vi "DataTranslation.vi"() -> (0 "error out":errorcluster)   [LabVIEW 2022 SP3]
uses:
  Sub_vis/Upload Data.ctl
  Globals/Meas_global.vi
  Data_Translation/Low levels/DtAinContinuous Folder/PolySubVIs/DtCreateAinChan.vi
  Data_Translation/Low levels/DtAinContinuous Folder/PolySubVIs/DtOLTimingSetInput.vi
  Data_Translation/Low levels/DtAinContinuous Folder/PolySubVIs/DtOLReadMultiple2D.vi
panel:
  out "Channels":string="0"
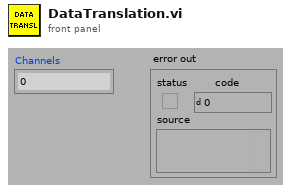
[diagram p1: front panel]
types:
  T1 = typedef "Analysis_info_cluster.ctl" = cluster{"Colour":u32, "Inst type":T2, "Inst name":string, "Symbol":string, "Code name":string, "Extra Info":string, "Inst Array":T3, "Extra Titles":string[], "Extra Values":string[], "U":dbl, "u^2":dbl, "u^3":dbl, "u^4":dbl, "Skew_u":dbl, "Kurt_u":dbl, "Sd Error in Mean":dbl, "% u'/U":dbl, "X":dbl, "Y":dbl, "Z":dbl, "Timescale integral Estimate":dbl, "Sd Error in Variance":dbl, "Calib File":path, "Calib Constants":dbl[], "Output Position":bool, "Stats":enum16{"None", "Basic", "Full"}, "Av Sampling Rate":dbl, "Av No of Samples":dbl, "Total Meas Time (s)":dbl, "ADAM Ch Name":string, "Max value":dbl, "Min value":dbl, "Req Sample Rate Hz":dbl, "Sync Delay Time (s)":dbl, "Ch No":i16, "Device":string, "Use Latest Calib":bool, "Port":string, "Metadata Ch Names":string[], "Metadata Ch Values":string[], "Label":string}
  T2 = typedef "Inst_type.ctl" = enum16{"Raw voltage", "Raw with zero offsetting", "Propeller anemometer", "Pressure Transducer", "Pitot-static tube", "Hot wire", "Cross wire 1", "Cross wire 2", "Generic Linear", "Generic Polynomial", "Generic BackPoly", "Fast FID", "Thermocouple", "Cold wire", "Pulsed Wire", "LDA Vel", "LDA Tran time", "LDA Arr time", "Microphone"}
  T3 = typedef "Instrument_Array.ctl" = enum16{"PWA", "LDA", "Analogue"}
  T4 = typedef "Device ID port info.ctl" = cluster{"Ch No":i16[], "Req Sampling Rate":dbl[], "Port":string, "Index":i32[]}
  T5 = typedef "Upload Data.ctl" = enum16{"Voltage Array", "Time Trace Cluster"}
  T6 = typedef "Setup.ctl" = enum16{"Run Program", "Show Setup", "Save Current Setup", "Setup Front Panel"}
  T7 = typedef "Rendezvous RefNum" = refnum<k1>
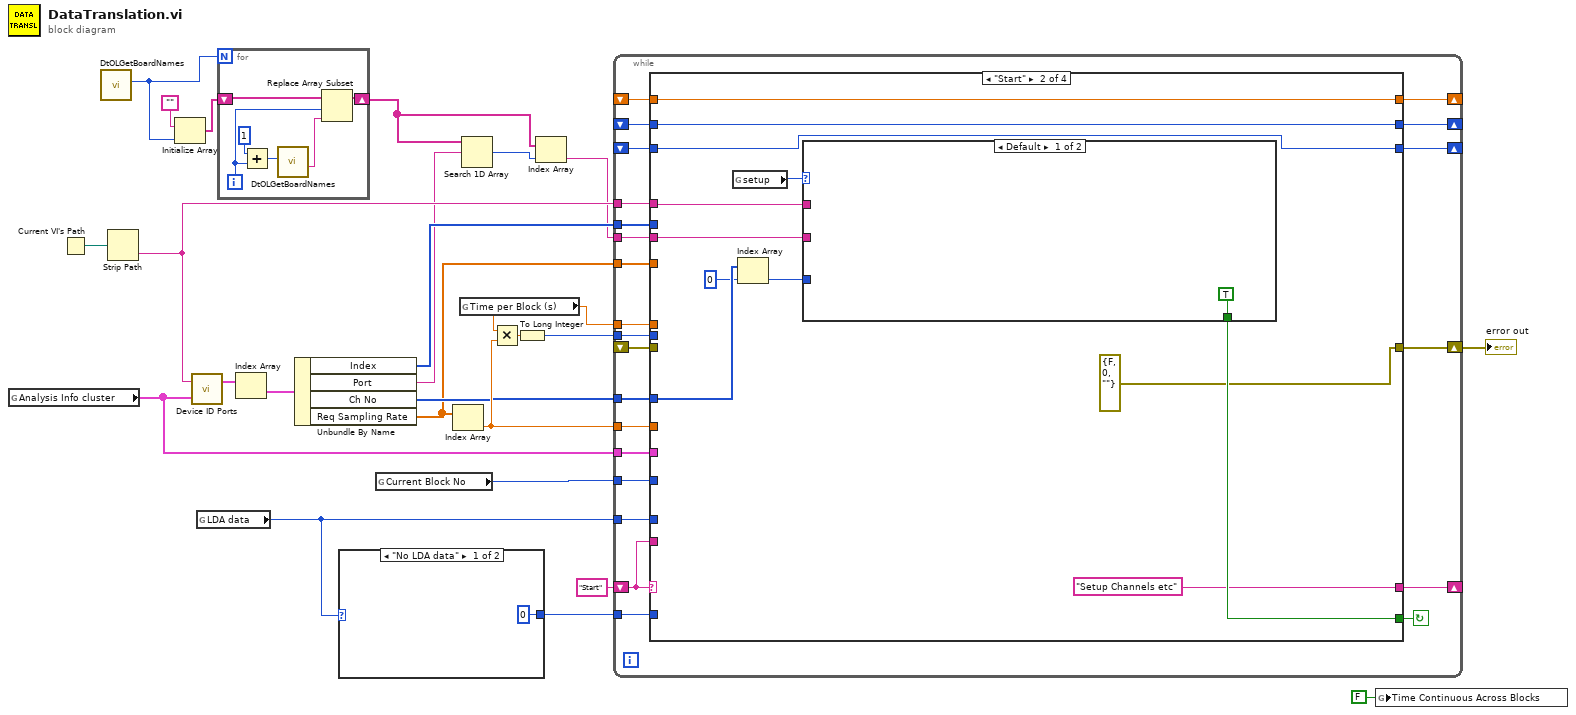
[diagram p0: block diagram]
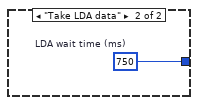
[diagram p2: hidden frame]
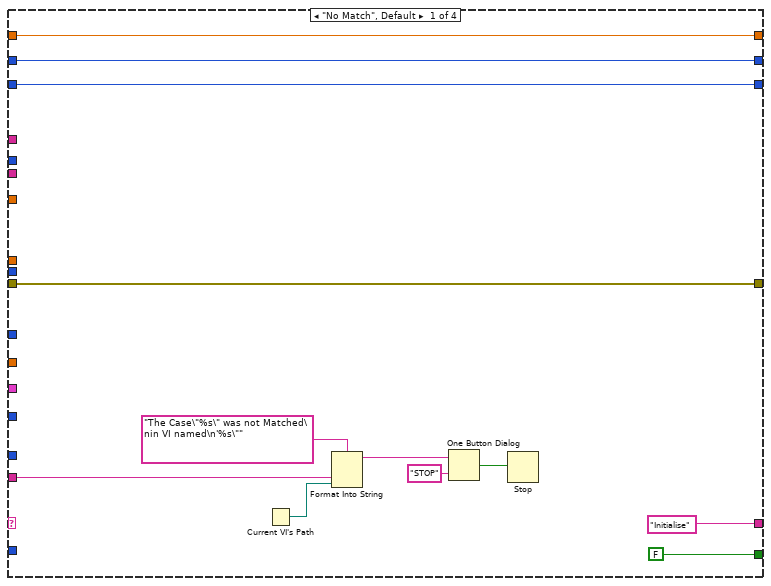
[diagram p3: hidden frame]
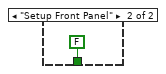
[diagram p4: hidden frame]
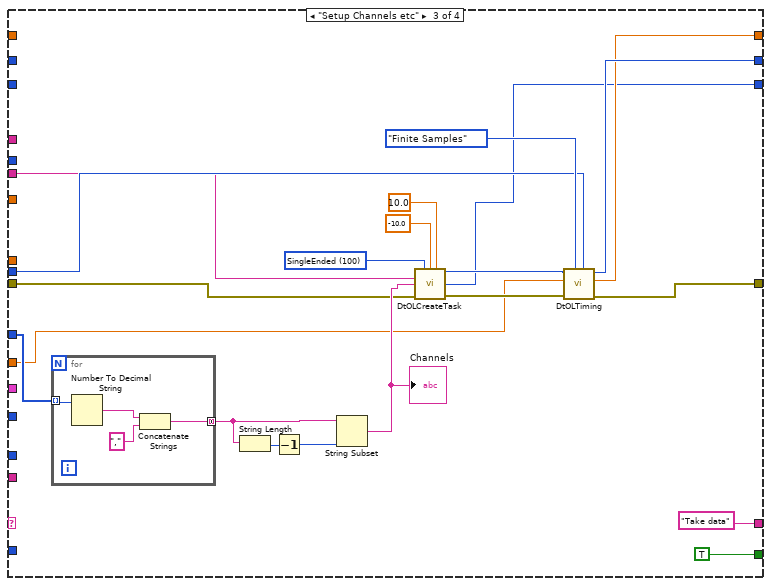
[diagram p5: hidden frame]
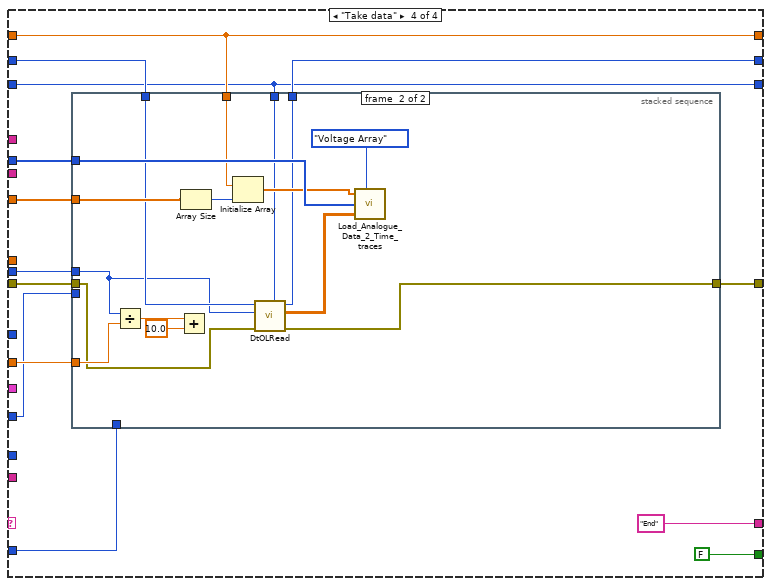
[diagram p6: hidden frame]
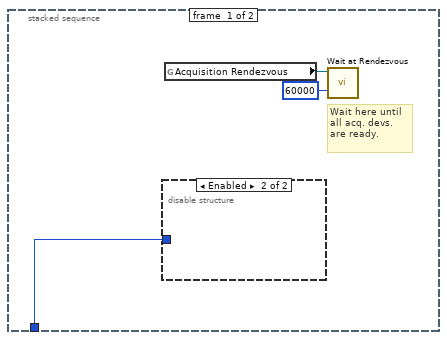
[diagram p7: hidden frame]
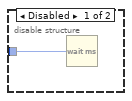
[diagram p8: hidden frame]
diagram:
  n1 = global read "Meas_global.vi" "Analysis Info cluster"() -> (w11:T1[])
  n2 = Current VI's Path() -> (path=w19:path)
  n3 = call "DtOLGetBoardNames.vi"() -> ("Number of boards"=w7:u32)  [unwired: 9 in, 2 out]
  n4 = Strip Path(path=w19) -> (name=w12:string)  [unwired: 1 out]
  n5 = Initialize Array("", w7) -> (w5:string[])
  n6 = call "Device ID Ports.vi"("Analysis Info cluster"=w11, "Device ID"=w12) -> ("Device port info"=w17:T4[])  [unwired: 1 out]
  n7 = global read "Meas_global.vi" "LDA data"() -> (w24:enum16{"No LDA data", "Take LDA data"})
  n8 = for {
    N: w7 -> [_]
    shift-right: [w28] -> w2
    shift-left: w5 -> [w29]
    i -> [w27]
    n9 = Add(x=1, y=w27) -> (x+y=w31:i32)
    n10 = call "DtOLGetBoardNames.vi"("Select Board"=w31) -> ("Board Name"=w26:string)  [unwired: 8 in, 2 out]
    n11 = Replace Array Subset(array=w29, new element=w26, index=w27) -> (w28:string[])
  }
  n12 = Index Array(array=w17) -> (element=w16:T4)  [unwired: 1 in]
  n13 = Unbundle By Name(w16) -> ("Index"=w15:i32[], "Port"=w4:string, "Ch No"=w14:i16[], "Req Sampling Rate"=w13:dbl[])
  n14 = case shown="\"No LDA data\"" w24 {
    tunnel: [u32 0 ("LDA wait time (ms)") w33] -> w22
    frame "No LDA data" {
    }
    frame "Take LDA data" {
      w33 = u32 750  # LDA wait time (ms)
    }
  }
  n15 = global read "Meas_global.vi" "Current Block No"() -> (w9:i32)
  n16 = Index Array(array=w13) -> (element=w18:dbl)  [unwired: 1 in]
  n17 = global read "Meas_global.vi" "Time per Block (s)"() -> (w10:dbl)
  n18 = Search 1D Array(1D array=w2, element=w4) -> (index of element=w3:i32)  [unwired: 1 in]
  n19 = Multiply(x=w10, y=w18) -> (x*y=w20:dbl)
  n20 = To Long Integer(number=w20) -> (32bit integer=w23:i32)
  n21 = Index Array(array=w2, index=w3) -> (element=w1:string)
  n22 = while {
    shift-left: "Start" -> [w56]
    shift-right: [w47] -> _
    shift-right: [w51] -> w21
    shift-left: _ -> [w55]
    tunnel: w18 -> [w54]
    tunnel: w23 -> [w53]
    tunnel: w9 -> [w52]
    shift-right: [w50] -> _
    shift-left: _ -> [w49]
    tunnel: w24 -> [w48]
    tunnel: w22 -> [w46]
    tunnel: w14 -> [w45]
    tunnel: w1 -> [w44]
    tunnel: w13 -> [w43]
    tunnel: w15 -> [w42]
    tunnel: w12 -> [w41]
    tunnel: w11 -> [w40]
    tunnel: w10 -> [w38]
    shift-right: [w37] -> _
    shift-left: _ -> [w36]
    shift-right: [w35] -> _
    shift-left: _ -> [w34]
    stop <- w39 continue-if-true
    n23 = case shown="\"Start\"" w56 {
      tunnel: [FALSE w73 TRUE FALSE] -> w39
      tunnel: ["Initialise" "Setup Channels etc" "Take data" "End"] -> w47
      tunnel: w56 -> [w63 _ _ _]
      tunnel: [w60 errorcluster {"status"=FALSE, "code"=0, "source"=""} ("error out") w90 w113] -> w51
      tunnel: w55 -> [w60 _ w89 w121]
      tunnel: w54 -> [_ _ w88 w118]
      tunnel: w53 -> [_ _ w86 w117]
      tunnel: w52 -> [_ _ _ w112]
      tunnel: [w59 w80 w85 w109] -> w50
      tunnel: w49 -> [w59 w80 _ w109]
      tunnel: w48 -> [_ _ _ _]
      tunnel: w46 -> [_ _ _ w116]
      tunnel: w45 -> [_ w76 w98 _]
      tunnel: w44 -> [_ w77 w83 _]
      tunnel: w43 -> [_ _ _ w115]
      tunnel: w42 -> [_ _ _ w114]
      tunnel: w41 -> [_ w79 _ _]
      tunnel: w40 -> [_ _ _ _]
      tunnel: w38 -> [_ _ _ _]
      tunnel: [w58 w70 w92 w110] -> w37
      tunnel: w36 -> [w58 w70 _ w111]
      tunnel: [w57 w69 w84 w108] -> w35
      tunnel: w34 -> [w57 w69 _ w108]
      frame "No Match", Default {
        n24 = Current VI's Path() -> (path=w62:path)
        n25 = Format Into String(format string="The Case\"%s\" was not Matched\nin VI named\n'%s\"" ("Format String"), w63, w62) -> (resulting string=w66:string)  [unwired: 2 in, 1 out]
        n26 = One Button Dialog(message=w66, button name ("OK")="STOP") -> (true=w64:bool)
        n27 = Stop(stop? (T)=w64) -> ()
      }
      frame "Start" {
        n28 = global read "Meas_global.vi" "setup"() -> (w78:T6)
        n29 = Index Array(array=w76, index=0) -> (element=w74:i16)
        n30 = case shown="Default" w78 {
          tunnel: w79 -> [_ _]
          tunnel: w77 -> [_ _]
          tunnel: w74 -> [_ _]
          tunnel: [TRUE FALSE] -> w73
          frame Default {
          }
          frame "Setup Front Panel" {
          }
        }
      }
      frame "Setup Channels etc" {
        w101 = 100 items=["SingleEnded"=100, "Differential"=101] ("Channel Type")
        n31 = for {
          tunnel: w98 -> [w107] mode=indexing
          tunnel: [w104] -> w97 mode=concatenating
          n32 = Number To Decimal String(number=w107) -> (decimal integer string=w106:string)  [unwired: 1 in]
          n33 = Concatenate Strings(w106, "," ("string")) -> (w104:string)
        }
        n34 = String Length(string=w97) -> (length=w96:i32)
        n35 = Decrement(x=w96) -> (x-1=w95:i32)
        n36 = String Subset(string=w97, length (rest)=w95) -> (substring=w94:string)  [unwired: 1 in]
        "Channels" <- w94
        n37 = call-poly "DtOLCreateTask.vi"("Channel Type"=w101, "Range Min"=-10.0, "Range Max"=10.0, "Board Name"=w83, "Channel"=w94, "error in (no error)"=w89) -> ("Task out"=w93:i32, "Actual Number of Channels"=w84:u32, "error out"=w91:errorcluster)  [unwired: 7 in]
        n38 = call-poly "DtOLTiming.vi"("Samples Per Channel"=w86, "Sample Mode"=enum16{"Finite Samples", "Continuous Samples"}."Finite Samples", "error in (no error)"=w91, "Sample Freq (Hz)"=w88, "Task in"=w93) -> ("error out"=w90:errorcluster, "Actual Sample Freq"=w85:dbl, "Task out"=w92:i32)  [unwired: 3 in, 1 out]
      }
      frame "Take data" {
        n39 = stacked-sequence {
          tunnel: w121 -> [_ w131]
          tunnel: w118 -> [_ w139]
          tunnel: w117 -> [_ w132]
          tunnel: [_ w128] -> w113
          tunnel: w116 -> [w124 _]
          tunnel: w115 -> [_ w137]
          tunnel: w114 -> [_ w138]
          tunnel: w112 -> [_ _]
          tunnel: w111 -> [_ w133]
          tunnel: [_ w130] -> w110
          tunnel: w109 -> [_ w127]
          tunnel: w108 -> [_ w126]
          frame #0 {
            # "Wait here until all acq. devs. are ready."
            n40 = disable-structure shown="Enabled" {
              disable-tunnel: w124 -> [w125 _]
              frame Disabled {
                n41 = Wait (ms)(milliseconds to wait=w125) -> ()  [unwired: 1 out]
              }
              frame Enabled {
              }
            }
            n42 = global read "Meas_global.vi" "Acquisition Rendezvous"() -> (w123:T7)
            n43 = call <vilib>:"Wait at Rendezvous.vi"("ms timeout (-1)"=60000, "rendezvous"=w123) -> ()  [unwired: 3 in, 3 out]
          }
          frame #1 {
            n44 = Divide(x=w132, y=w139) -> (x/y=w141:dbl)
            n45 = Add(x=w141, y=10.0) -> ()  [unwired: 1 out]
            n46 = Array Size(array=w137) -> (size(s)=w136:i32)
            n47 = Initialize Array(w127, w136) -> (w135:dbl[])
            n48 = call-poly "DtOLRead.vi"("Number Chan to Read"=w126, "error in (no error)"=w131, "Samples Per Channel"=w132, "Task in"=w133) -> ("error out"=w128:errorcluster, "2D Data out"=w129:dbl[][], "Task out"=w130:i32)  [unwired: 3 in, 2 out]
            n49 = call "Load_Analogue_Data_2_Time_traces.vi"("Sampling Rate (Hz)"=w135, "Mode"=Upload_Data."Voltage Array", "Index"=w138, "Voltage Array"=w129) -> ()  [unwired: 3 in]
          }
        }
      }
    }
  }
  "error out" <- w21
  n50 = global write "Meas_global.vi" "Time Continuous Across Blocks"(FALSE ("Time Continuous Across Blocks")) -> ()
